vi "RetryOnError.vi"(8 "error in (no error)":errorcluster, 11 "Error Msg":string) -> (0 "error out":errorcluster, 4 "Retry":bool)   [LabVIEW 2014]
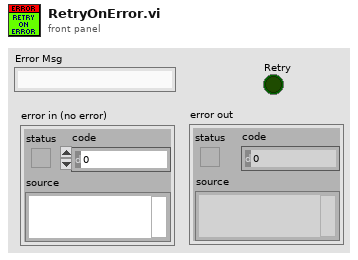
[diagram p1: front panel]
types:
  T1 = enum16{"Left Button", "Center Button", "Right Button", "Window Close"}
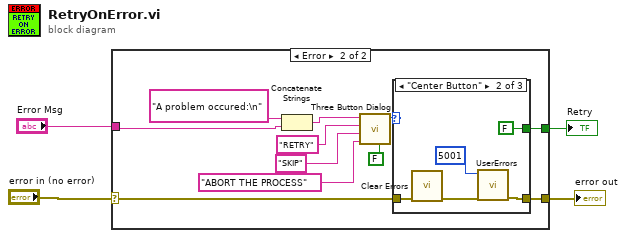
[diagram p0: block diagram]
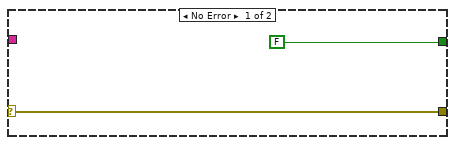
[diagram p2: hidden frame]
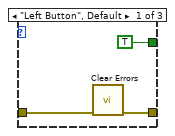
[diagram p3: hidden frame]
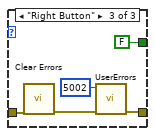
[diagram p4: hidden frame]
diagram:
  n1 = case shown="Error" "error in (no error)" {
    selector: "error in (no error)" -> [w5 w9]
    tunnel: [FALSE w7] -> w3
    tunnel: [w5 w8] -> w2
    tunnel: "Error Msg" -> [_ w16]
    frame No Error {
    }
    frame Error {
      n2 = Concatenate Strings("A problem occured:\n" ("message"), w16) -> (w15:string)
      n3 = call <vilib>:"Three Button Dialog.vi"("Allow user to close window? (TRUE)"=FALSE, "Right Button Text (\"Cancel\")"="ABORT THE PROCESS" ("F button name (\"Cancel\")"), "Center Button Text (\"No\")"="SKIP" ("T button name (\"OK\")"), "Left Button Text (\"Yes\")"="RETRY" ("T button name (\"OK\")"), "message"=w15) -> ("Which Button?"=w10:T1)  [unwired: 6 in]
      n4 = case shown="\"Center Button\"" w10 {
        tunnel: w9 -> [w19 w25 w27]
        tunnel: [w18 w24 w29] -> w8
        tunnel: [TRUE FALSE FALSE] -> w7
        frame "Left Button", Default {
          n5 = call <vilib>:"Clear Errors.vi"("error in (no error)"=w19) -> ("error out"=w18:errorcluster)  [unwired: 5 in, 1 out]
        }
        frame "Center Button" {
          n6 = call <vilib>:"Clear Errors.vi"("error in (no error)"=w25) -> ("error out"=w21:errorcluster)  [unwired: 5 in, 1 out]
          n7 = call "UserErrors.vi"("error in (no error)"=w21, "[error code] (0)"=5001) -> ("error out"=w24:errorcluster)  [unwired: 9 in]
        }
        frame "Right Button" {
          n8 = call <vilib>:"Clear Errors.vi"("error in (no error)"=w27) -> ("error out"=w26:errorcluster)  [unwired: 5 in, 1 out]
          n9 = call "UserErrors.vi"("error in (no error)"=w26, "[error code] (0)"=5002) -> ("error out"=w29:errorcluster)  [unwired: 9 in]
        }
      }
    }
  }
  "error out" <- w2
  "Retry" <- w3
